vi "LVProjectShortcut_Command.vi"(8 "error in":errorcluster, 10 "Command":string, 11 "Object":T1) -> (0 "error out":errorcluster)   [LabVIEW 2017]
uses:
  <resource>/Framework/Providers/API/ItemRef.ctl
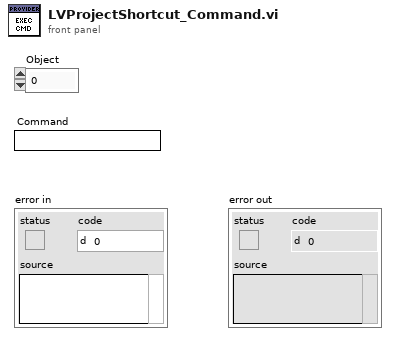
[diagram p1: front panel]
types:
  T1 = typedef "ItemRef.ctl" = u64
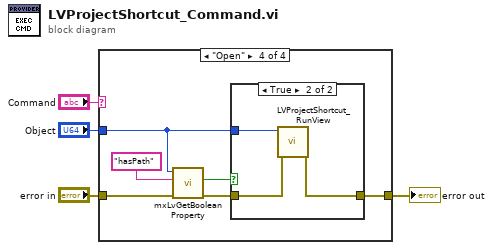
[diagram p0: block diagram]
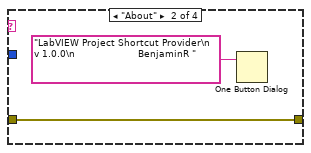
[diagram p3: hidden frame]
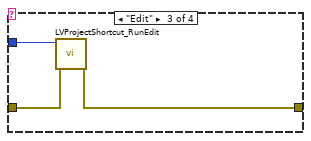
[diagram p4: hidden frame]
diagram:
  n1 = case shown="\"Open\"" "Command" {
    tunnel: "Object" -> [_ _ w10 w12]
    tunnel: "error in" -> [w5 w6 w9 w15]
    tunnel: [w5 w6 w8 w13] -> w1
    frame Default {
    }
    frame "About" {
      n2 = One Button Dialog(message="LabVIEW Project Shortcut Provider\n                        v 1.0.0\n                     BenjaminR ") -> ()  [unwired: 1 in, 1 out]
    }
    frame "Edit" {
      n3 = call "LVProjectShortcut_RunEdit.vi"("error in (no error)"=w9, "Object"=w10) -> ("error out"=w8:errorcluster)  [unwired: 9 in]
    }
    frame "Open" {
      n4 = call <resource>:"mxLvGetBooleanProperty.vi"("error in"=w15, "Tag"="hasPath", "Item"=w12) -> ("error out"=w14:errorcluster, "Value"=w11:bool)  [unwired: 6 in, 1 out]
      n5 = case shown="True" w11 {
        tunnel: w14 -> [w17 w19]
        tunnel: [w17 w18] -> w13
        tunnel: w12 -> [_ w20]
        frame False {
        }
        frame True {
          n6 = call "LVProjectShortcut_RunView.vi"("error in (no error)"=w19, "Object"=w20) -> ("error out"=w18:errorcluster)  [unwired: 9 in]
        }
      }
    }
  }
  "error out" <- w1
